vi "Hardware Globals.vi"() -> ()   [LabVIEW 2018]
panel:
  in  "Zaber VISA":refnum<visa-resource-name>
  in  "Motor Conv":dbl format="%#_8g"
  in  "Pump Cnts":i32
  in  "COM ports in use":string[](array[string])
  in  "Servo Ctrlr":refnum<visa-resource-name>
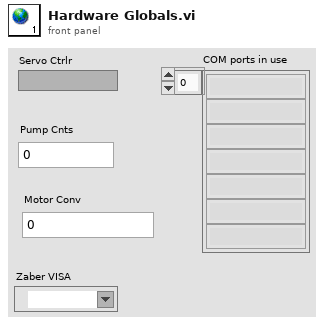
[diagram p1: front panel]
diagram:
